vi "Revision.vi"() -> ()   [LabVIEW 2020]
panel:
  out "Revision":i64
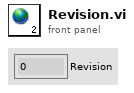
[diagram p1: front panel]
diagram:
